vi "scanallchannels_test_carac.vi"(0 "Instrument VISA in":T1={"AWG VISA"="81160A", "Oscilloscope  VISA "="DSO80204B", "Integration Board IP"="172.16.7.43", "connection ID"=refnum, "report out"=refnum, "report file path"=path "D:/CTA/LevelTriggerBoardTest/TestsData/sumtrigger_delay"}, 2 "Save test data":bool=TRUE, 5 "Channels values":i32[](array[numeric])=[0, 1, 2], 7 "Channels init":i32[](array[numeric])=[2000, 2000, 2000, 2000, 5, 6], 9 "Cycles Burst":i32=10000, 11 "error in":errorcluster, 12 "L1 version":bool) -> (4 "Instrument VISA out":T1={"AWG VISA"="81160A", "Oscilloscope  VISA "="DSO80204B", "Integration Board IP"="172.16.7.43", "connection ID"=refnum, "report out"=refnum, "report file path"=path "D:/CTA/LevelTriggerBoardTest/TestsData/sumtrigger_delay"}, 10 "Channels values":i32[](array[numeric])=[0, 1, 2, 3, 5, 6, 7], 15 "error out":errorcluster={"status"=TRUE, "code"=8, "source"=""})   [LabVIEW 2009]
doc: "This VI does a DTs calibration for Majority Trigger boards."
uses:
  <vilib>/Utility/NIReport.llb/NI_report.lvclass
  <vilib>/Utility/NIReport.llb/HTML/NI_HTML.lvclass
  <instrlib>/Agilent 81150/Agilent 81150.lvlib
panel:
  in  "Channels clip":i32[](array[numeric])=[0, 1, 2, 3, 4, 5, 6]
  out "L1  50%":dbl[][][][](array[numeric])
  in  "Voltages values":dbl[](array[numeric])=[0.05, 0.1, 0.2, 0.3, 0.4, 0.5, 0.6, 0.7, 0.8, 0.9, 1.0, 1.1, 1.2, 1.3, 1.4, 1.5, 2.0, 2.5]
  out "report file path":path=path "D:/CTA/LevelTriggerBoardTest/TestsData/sumtrigger_delay"
  out "IPR_Address":i32=23
  out "L1 Address":i32=17
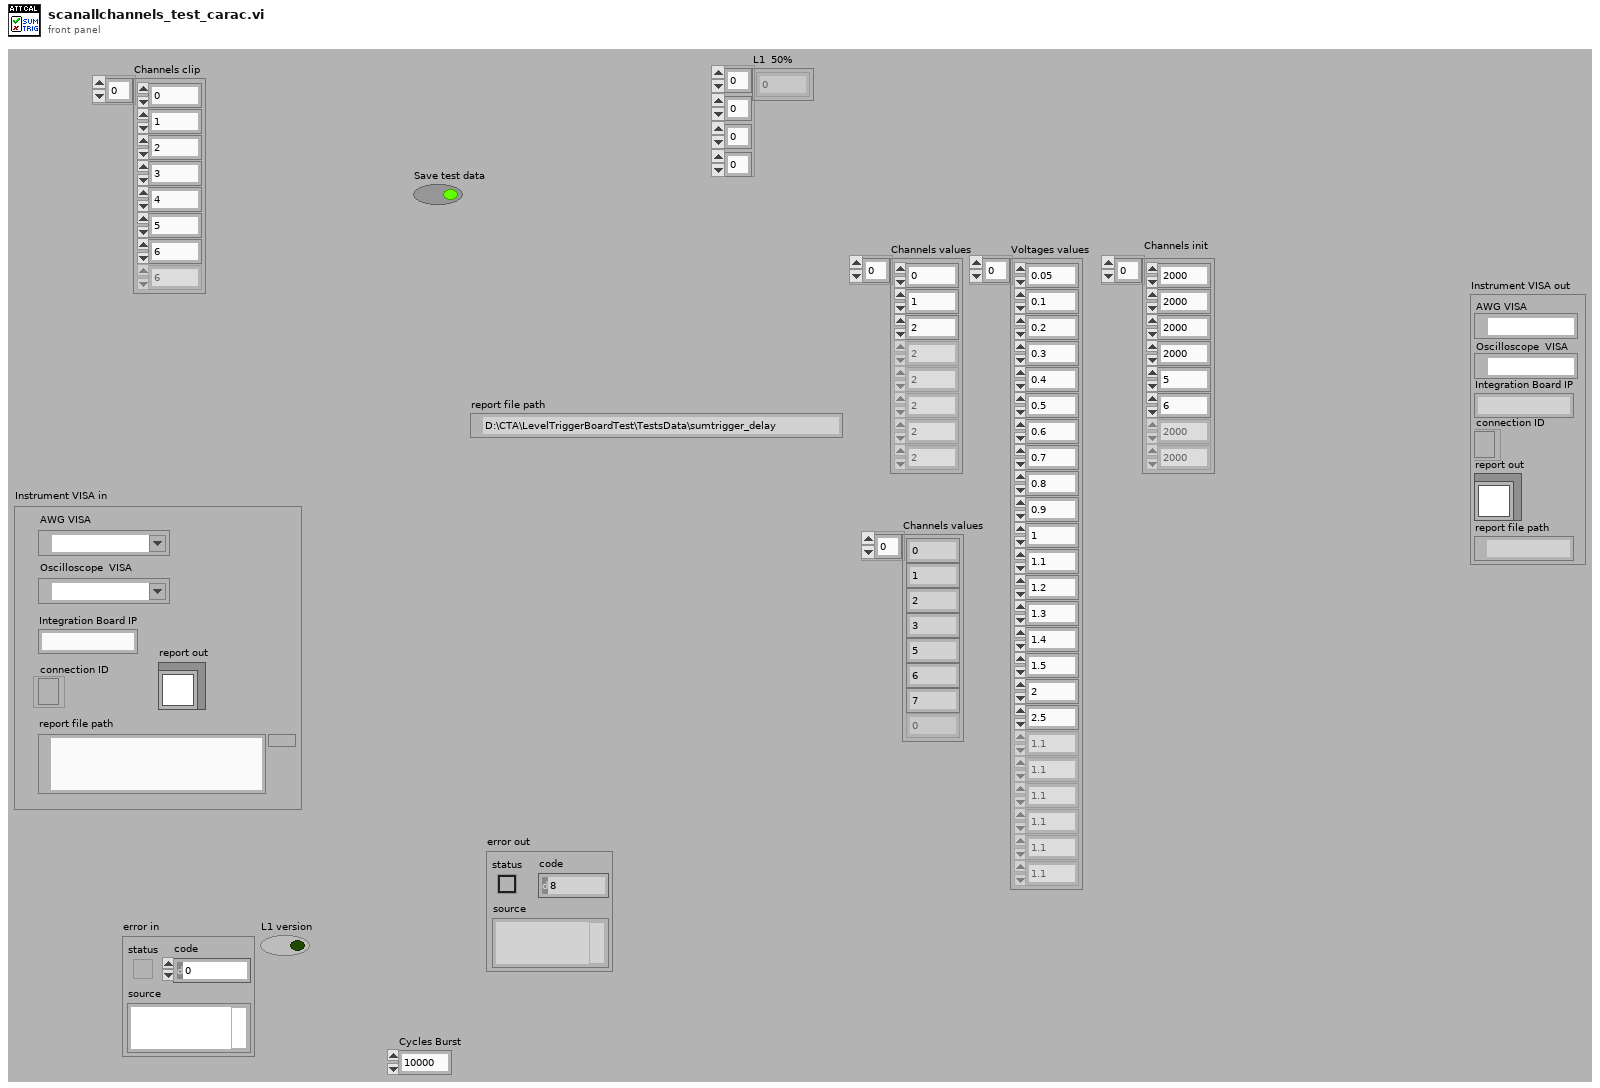
[diagram p1: front panel]
types:
  T1 = cluster{"AWG VISA":refnum<visa-resource-name>, "Oscilloscope  VISA ":refnum<visa-resource-name>, "Integration Board IP":string, "connection ID":refnum<k5>, "report out":refnum<class "NI_report.lvclass">, "report file path":path}
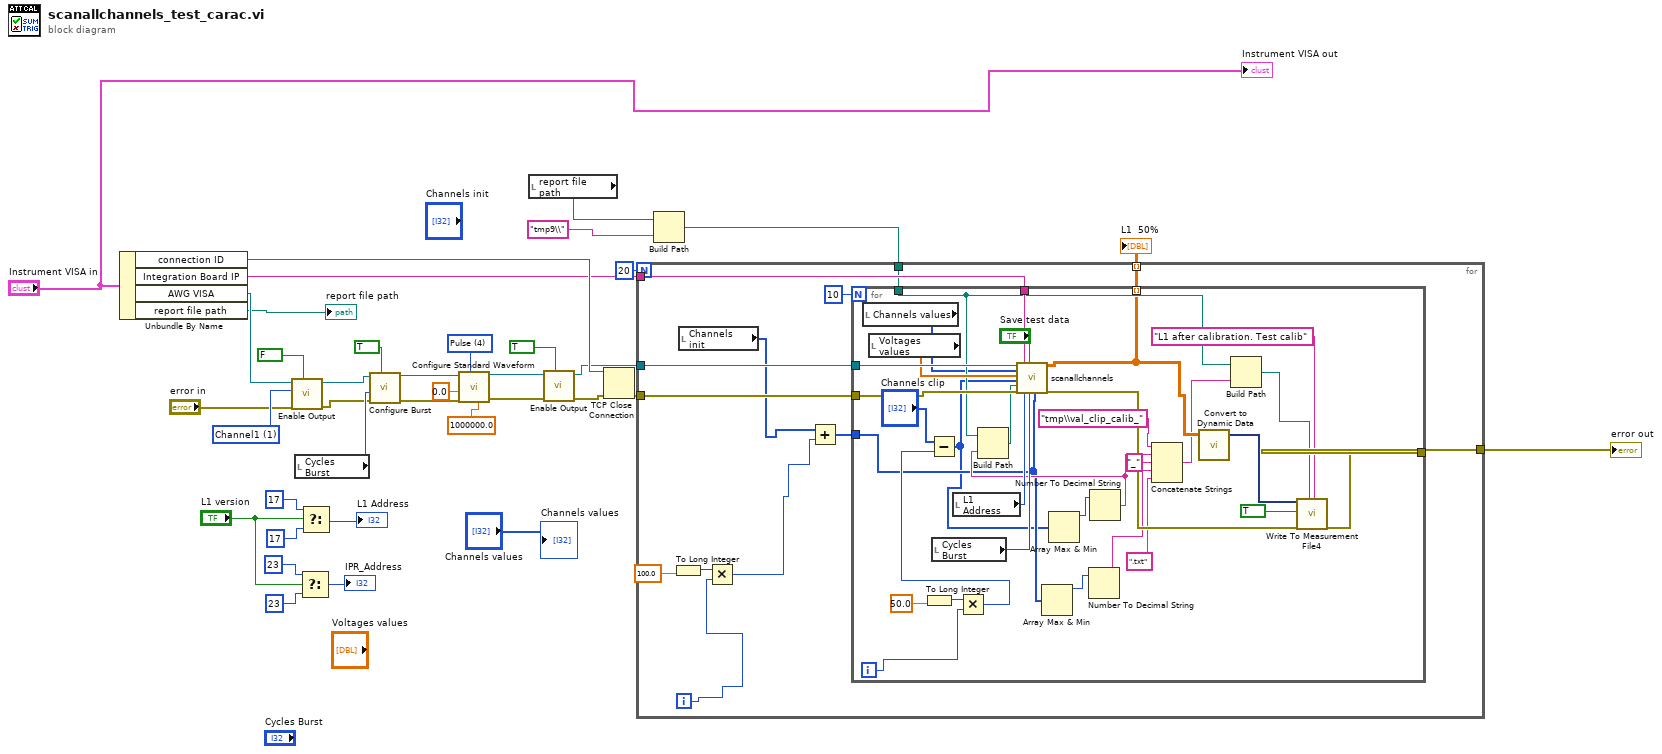
[diagram p0: block diagram]
diagram:
  w29 = u16 4 items=["Sine", "Square", "Ramp Up", "Ramp Down", "Pulse", "Noise", "DC"] ("Waveform (0: Sine)")
  w36 = u16 1 items=["Channel1"=1, "Channel2"=2] ("Channel (1: Channel1)")
  n1 = Unbundle By Name("Instrument VISA in") -> ("connection ID"=w15:refnum<k5>, "Integration Board IP"=w7:string, "AWG VISA"=w30:refnum<visa-resource-name>, "report file path"=→"report file path":path)
  n2 = call <instrlib>:"Enable Output.vi"("Enable Output (T: Enable)"=FALSE, "error in (no error)"="error in", "Channel (1: Channel1)"=w36, "VISA resource name"=w30) -> ("error out"=w14:errorcluster, "VISA resource name out"=w13:refnum<visa-resource-name>)  [unwired: 6 in]
  n3 = local read "Cycles Burst"() -> (w17:i32)
  n4 = Select(t=23 ("Address"), s="L1 version", f=23 ("Address")) -> (s? t:f=→"IPR_Address":i32)
  n5 = Select(t=17 ("Address"), s="L1 version", f=17 ("Address")) -> (s? t:f=→"L1 Address":i32)
  n6 = call <instrlib>:"Configure Burst.vi"("Enable Burst (F: Disable)"=TRUE, "error in (no error)"=w14, "Burst Count (2)"=w17, "VISA resource name"=w13) -> ("error out"=w26:errorcluster, "VISA resource name out"=w27:refnum<visa-resource-name>)  [unwired: 6 in]
  n7 = call <instrlib>:"Configure Standard Waveform.vi"("Frequency (1000.0 Hz)"=1000000.0, "Waveform (0: Sine)"=w29, "error in (no error)"=w26, "Amplitude (1.0 Vpp)"=0.0, "VISA resource name"=w27) -> ("error out"=w25:errorcluster, "VISA resource name out"=w24:refnum<visa-resource-name>)  [unwired: 5 in]
  n8 = local read "report file path"() -> (w11:path)
  n9 = call <instrlib>:"Enable Output.vi"("Enable Output (T: Enable)"=TRUE, "error in (no error)"=w25, "VISA resource name"=w24) -> ("error out"=w16:errorcluster, "VISA resource name out"=w8:refnum<visa-resource-name>)  [unwired: 7 in]
  n10 = TCP Close Connection(connection ID=w15, error in (no error)=w16) -> (error out=w9:errorcluster)  [unwired: 1 in, 1 out]
  n11 = Build Path(base path=w11, name or relative path="tmp9\\") -> (appended path=w4:path)
  n12 = for {
    N: 20 -> [_]
    tunnel: w9 -> [w50]
    tunnel: w8 -> [w49]
    tunnel: w7 -> [w48]
    tunnel: w4 -> [w47]
    tunnel: [w46] -> w2 mode=indexing
    tunnel: [w45] -> w3
    i -> [w39]
    n13 = To Long Integer(number=100.0 ("x")) -> (32bit integer=w42:i32)
    n14 = local read "Channels init"() -> (w40:i32[])
    n15 = Multiply(x=w42, y=w39) -> (x*y=w38:i32)
    n16 = Add(x=w40, y=w38) -> (x+y=w43:i32[])
    n17 = for {
      N: 10 -> [_]
      tunnel: [w73] -> w45
      tunnel: w50 -> [w82]
      tunnel: w49 -> [w81]
      tunnel: w48 -> [w80]
      tunnel: w47 -> [w69]
      tunnel: [w68] -> w46 mode=indexing
      tunnel: w43 -> [w54]
      i -> [w60]
      n18 = local read "Channels values"() -> (w63:i32[])
      n19 = local read "Voltages values"() -> (w79:dbl[])
      n20 = To Long Integer(number=50.0 ("x")) -> (32bit integer=w62:i32)
      n21 = local read "Cycles Burst"() -> (w77:i32)
      n22 = local read "L1 Address"() -> (w78:i32)
      n23 = Multiply(x=w62, y=w60) -> (x*y=w58:i32)
      n24 = Subtract(x="Channels clip", y=w58) -> (x-y=w53:i32[])
      n25 = Array Max & Min(array=w54) -> (max value=w51:i32)  [unwired: 3 out]
      n26 = Array Max & Min(array=w53) -> (max value=w52:i32)  [unwired: 3 out]
      n27 = Number To Decimal String(number=w51) -> (decimal integer string=w56:string)  [unwired: 1 in]
      n28 = Number To Decimal String(number=w52) -> (decimal integer string=w65:string)  [unwired: 1 in]
      n29 = Build Path(base path=w69, name or relative path=w65) -> (appended path=w75:path)
      n30 = call "scanallchannels.vi"("VISA resource name out"=w81, "nm ch"=w63, "Voltages values"=w79, "Init ch value"=w53, "base path"=w75, "error in"=w82, "Integration Board IP"=w80, "L1 Address"=w78, "Save test data"="Save test data", "Ch burst"=w77, "vclip"=w54) -> ("L1  50%"=w68:dbl[][], "error out"=w74:errorcluster)  [unwired: 6 in, 1 out]
      n31 = Concatenate Strings("tmp\\val_clip_calib_" ("name or relative path"), w65, "_" ("string"), w56, ".txt" ("string")) -> (w66:string)
      n32 = call "Convert to Dynamic Data"("2D Array"=w68) -> ("Dynamic Data Type"=w72:dynamicdata)  [unwired: 3 in]
      n33 = Build Path(base path=w69, name or relative path=w66) -> (appended path=w70:path)
      n34 = call "Write To Measurement File4"("Signals"=w72, "Enable"=TRUE, "error in (no error)"=w74, "Filename"=w70, "Comment"="L1 after calibration. Test calib") -> ("error out"=w73:errorcluster)  [unwired: 12 in, 2 out]
    }
  }
  "error out" <- w3
  "L1  50%" <- w2
  "Instrument VISA out" <- "Instrument VISA in"
  "Channels values" <- "Channels values"
